vi "E7_30_READ_BUFFER_2.vi"(8 "error in":T6, 11 "DriverConnect in":T1={"InterfaceType"=enum."VISA", "OpenedSession"="", "InterfaceSettings"={"Interface"=enum."RS232", "EOS 4 read"=enum."LF (\\n)", "EOS 4 write"=enum."LF (\\n)", "TMO, ms"=10000, "Sett"=variant(cluster{"Baud Rate":u32, "Data Bits":u16, "Parity":u16, "Stop Bits":u16, "Flow Control":u16, "Eho":bool} {"Baud Rate"=75, "Data Bits"=0, "Parity"=0, "Stop Bits"=0, "Flow Control"=0, "Eho"=FALSE})}}) -> (0 "error out":T6, 3 "DriverConnect out":T1={"InterfaceType"=enum."VISA", "OpenedSession"="", "InterfaceSettings"={"Interface"=enum."RS232", "EOS 4 read"=enum."LF (\\n)", "EOS 4 write"=enum."LF (\\n)", "TMO, ms"=10000, "Sett"=variant(cluster{"Baud Rate":u32, "Data Bits":u16, "Parity":u16, "Stop Bits":u16, "Flow Control":u16, "Eho":bool} {"Baud Rate"=75, "Data Bits"=0, "Parity"=0, "Stop Bits"=0, "Flow Control"=0, "Eho"=FALSE})}}, 5 "String from device out":string)   [LabVIEW 2018]
uses:
  MOKO_LabViewLibrary/MokoLowLevel/MokoLowLovelControl/MLLC_Error.ctl
  MOKO_LabViewLibrary/MokoLowLevel/MokoLowLovelControl/MLLC_ConnectCluster.ctl
  MOKO_LabViewLibrary/MokoLowLevel/MokoLowLovelControl/MLLC_InterfaceType.ctl
  MOKO_LabViewLibrary/MokoLowLevel/MokoLowLovelControl/MLLC_OpenedSession.ctl
  MOKO_LabViewLibrary/MokoLowLevel/MokoLowLovelControl/MLLC_InterfaceSettings.ctl
  MOKO_LabViewLibrary/MokoLowLevel/MokoLowLovelControl/MLLC_InterfaceKind.ctl
  MOKO_LabViewLibrary/MokoLowLevel/MokoLowLovelControl/MLLC_Rs232Settings.ctl
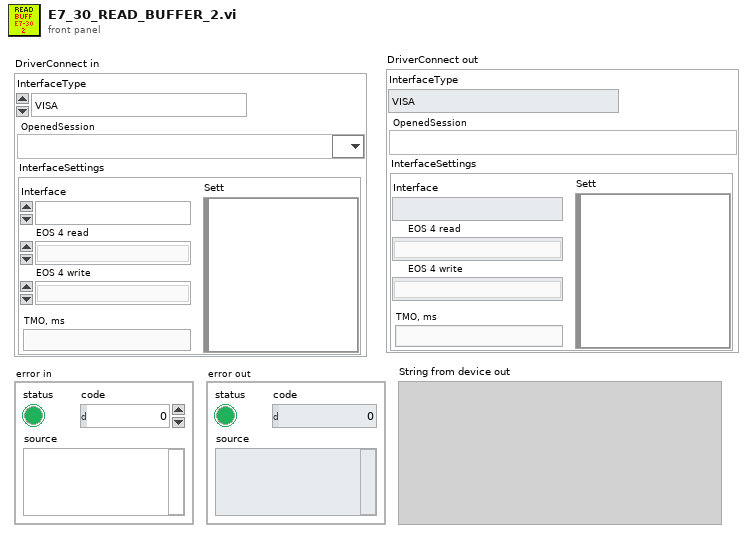
[diagram p1: front panel]
types:
  T1 = typedef "MLLC_ConnectCluster.ctl" = cluster{"InterfaceType":T2, "OpenedSession":T3, "InterfaceSettings":T4}
  T2 = typedef "MLLC_InterfaceType.ctl" = enum16{"VISA", "Prologix USB-GPIB"}
  T3 = typedef "MLLC_OpenedSession.ctl" = refnum<visa-resource-name>
  T4 = typedef "MLLC_InterfaceSettings.ctl" = cluster{"Interface":T5, "EOS 4 read":enum16{"Default (=EOS 4 write)", "CR (\\r)", "LF (\\n)", "None"}, "EOS 4 write":enum16{"CR+LF (\\r\\n)", "CR (\\r)", "LF (\\n)", "None"}, "TMO, ms":i32, "Sett":variant}
  T5 = typedef "MLLC_InterfaceKind.ctl" = enum16{"RS232", "GPIB", "USB", "Ethernet", "another"}
  T6 = typedef "MLLC_Error.ctl" = errorcluster
  T7 = typedef "MLLC_Rs232Settings.ctl" = cluster{"Baud Rate":u32, "Data Bits":u16, "Parity":u16, "Stop Bits":u16, "Flow Control":u16, "Eho":bool, "Address":dbl}
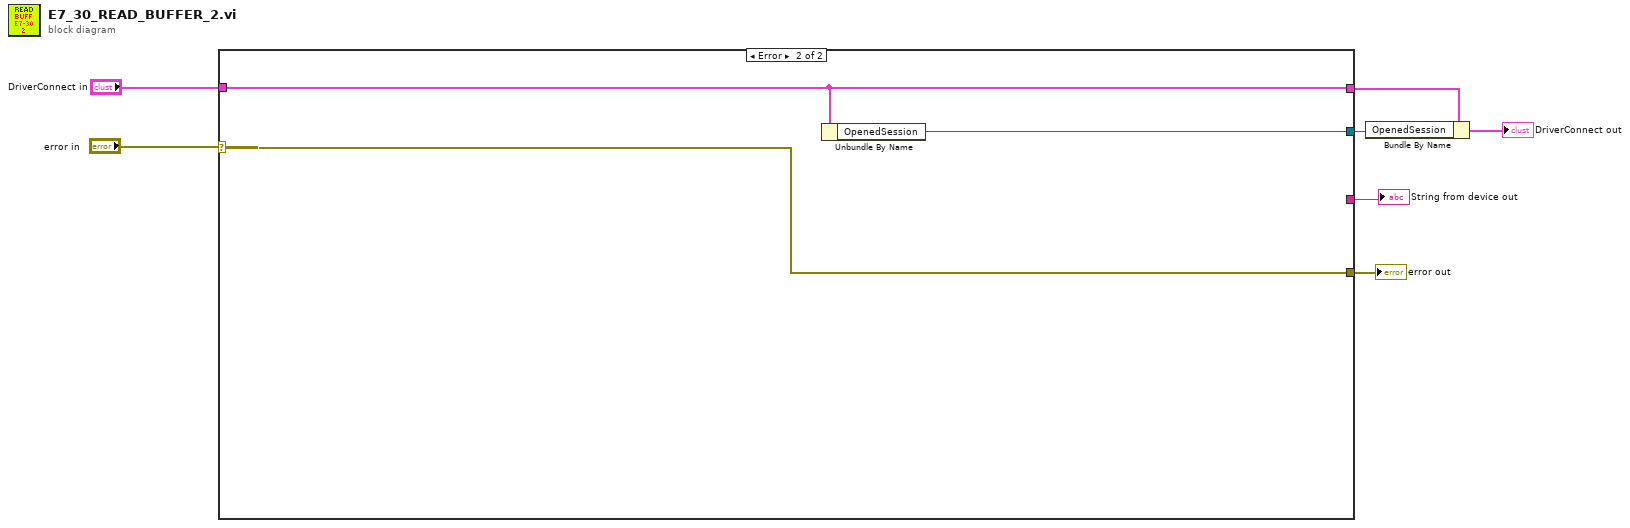
[diagram p0: block diagram]
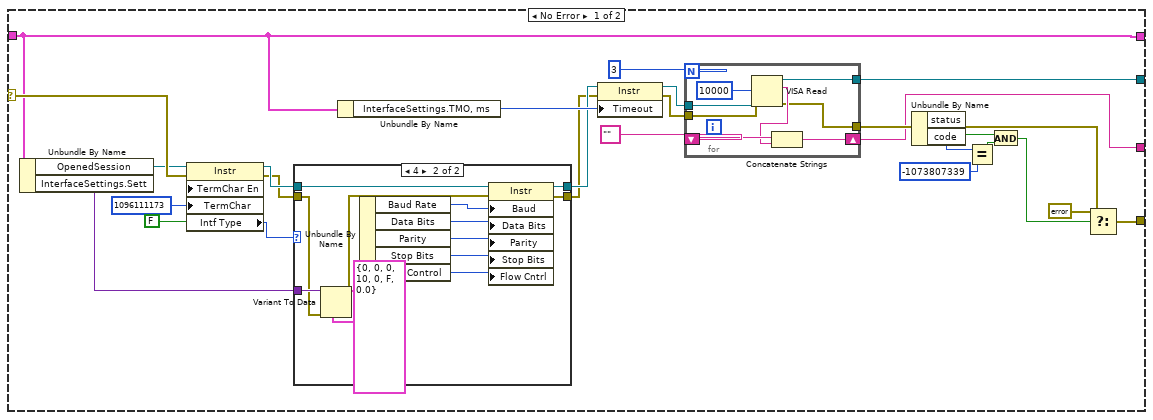
[diagram p2: hidden frame]
diagram:
  n1 = case shown="Error" "error in" {
    selector: "error in" -> [w25 w59]
    tunnel: [w13 _] -> w7
    tunnel: [w32 w59] -> w6
    tunnel: [w14 w57] -> w3
    tunnel: [w8 w58] -> w2
    tunnel: "DriverConnect in" -> [w8 w58]
    frame No Error {
      n2 = Unbundle By Name(w8) -> ("OpenedSession"=w9:T3, "InterfaceSettings.Sett"=w22:variant)
      n3 = property class="Instr"(reference=w9, error in=w25, "TermChar En"=FALSE ("Message Based Settings:Termination Character Enable"), "TermChar"=u64 1096111173 ("Message Based Settings:Termination Character")) -> (reference out=w24:T3, error out=w23:errorcluster, "Intf Type"=w18:u16)
      n4 = case shown="4" w18 {
        tunnel: [w43 w52] -> w19
        tunnel: w24 -> [w43 w53]
        tunnel: [w42 w44] -> w11
        tunnel: w23 -> [w42 w55]
        tunnel: w22 -> [_ w56]
        frame 0, Default {
        }
        frame 4 {
          n5 = Variant To Data(error in=w55, type=T7 {"Baud Rate"=0, "Data Bits"=0, "Parity"=0, "Stop Bits"=10, "Flow Control"=0, "Eho"=FALSE, "Address"=0.0} ("Cluster"), Variant=w56) -> (data=w50:T7, error out=w54:errorcluster)
          n6 = Unbundle By Name(w50) -> ("Baud Rate"=w49:u32, "Data Bits"=w45:u16, "Parity"=w46:u16, "Stop Bits"=w47:u16, "Flow Control"=w48:u16)
          n7 = property class="Instr"(reference=w53, error in=w54, "Baud"=w49, "Data Bits"=w45, "Parity"=w46, "Stop Bits"=w47, "Flow Cntrl"=w48) -> (reference out=w52:T3, error out=w44:errorcluster)
        }
      }
      n8 = Unbundle By Name(w8) -> ("InterfaceSettings.TMO, ms"=w20:i32)
      n9 = property class="Instr"(reference=w19, error in=w11, "Timeout"=w20) -> (reference out=w17:T3, error out=w16:errorcluster)
      n10 = for {
        N: 3 ("length (rest)") -> [_]
        shift-right: [w37] -> w13
        shift-left: "" ("read buffer") -> [w36]
        tunnel: w17 -> [w40]
        tunnel: w16 -> [w39]
        tunnel: [w34] -> w15
        tunnel: [w38] -> w14
        n11 = VISA Read(VISA resource name=w40, byte count=u32 10000, error in (no error)=w39) -> (VISA resource name out=w38:T3, read buffer=w35:string, error out=w34:errorcluster)  [unwired: 1 out]
        n12 = Concatenate Strings(w36, w35) -> (w37:string)
      }
      n13 = Unbundle By Name(w15) -> ("status"=w28:bool, "code"=w31:i32)
      n14 = Equal?(x=w31, y=-1073807339) -> (x = y?=w29:bool)
      n15 = And(x=w28, y=w29) -> (x .and. y?=w27:bool)
      n16 = Select(t=errorcluster {"status"=FALSE, "code"=0, "source"=""} ("error IO"), s=w27, f=w15) -> (s? t:f=w32:errorcluster)
    }
    frame Error {
      n17 = Unbundle By Name(w58) -> ("OpenedSession"=w57:T3)
    }
  }
  "String from device out" <- w7
  "error out" <- w6
  n18 = Bundle By Name(cluster=w2, "OpenedSession"=w3) -> (→"DriverConnect out":T1)
